vi "ShowTableResults.vi"(0 "session in":refnum<k35>, 7 "Data Result":T1(array[cluster]), 11 "error in":errorcluster) -> (4 "session out":refnum<k35>, 15 "error out":errorcluster)   [LabVIEW 2023]
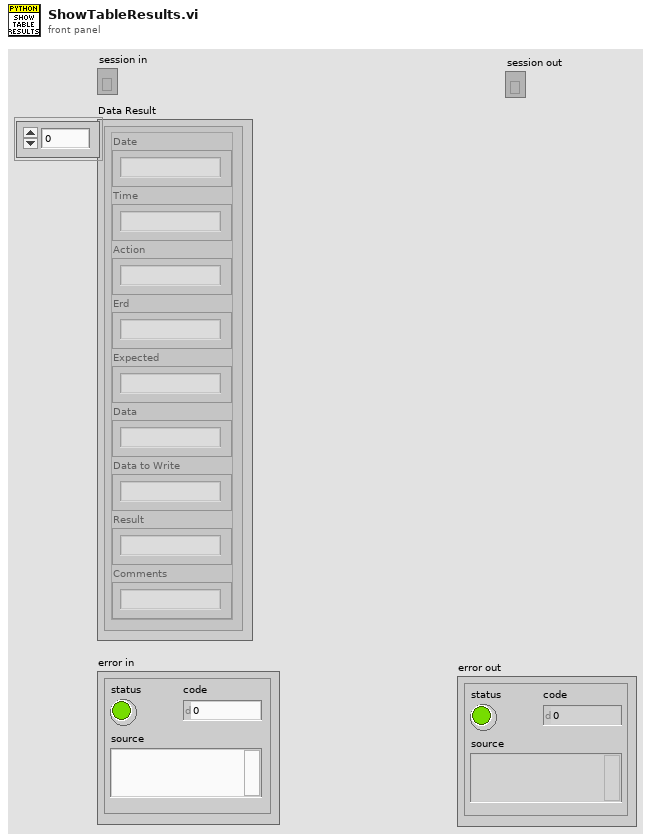
[diagram p1: front panel]
types:
  T1 = cluster{"Date":string, "Time":string, "Action":string, "Erd":string, "Expected":string, "Data":string, "Data to Write":string, "Result":string, "Comments":string}[]
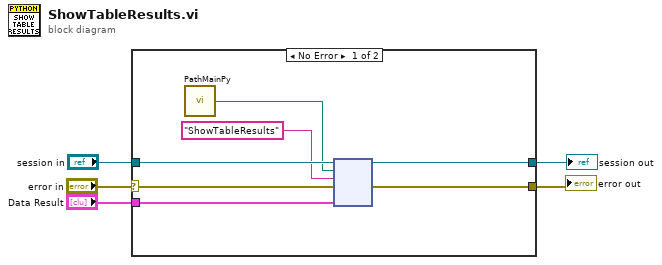
[diagram p0: block diagram]
diagram:
  n1 = case shown="No Error" "error in" {
    selector: "error in" -> [w9 w13]
    tunnel: "session in" -> [w12 w14]
    tunnel: [w11 w14] -> w2
    tunnel: [w10 w13] -> w3
    tunnel: "Data Result" -> [w6 _]
    frame No Error {
      n2 = call "PathMainPy.vi"() -> ("path"=w8:path)  [unwired: 15 in]
      n3 = node(w12, w8, "ShowTableResults" ("function name"), w9, w6) -> (w11:refnum<k35>, w10:errorcluster)  [unwired: 3 in, 2 out]
    }
    frame Error {
    }
  }
  "error out" <- w3
  "session out" <- w2
